vi "DrawChampionsScreen.vi"(8 "error in (no error)":errorcluster, 11 "SnakeGame in":refnum<class "SnakeGame.lvclass">) -> (0 "error out":errorcluster, 3 "SnakeGame out":refnum<class "SnakeGame.lvclass">)   [LabVIEW 2019, in "RT_Game.lvlib" / "SnakeGame.lvclass"]
uses:
  SnakeGame.lvclass
  Engine/Engine.lvclass
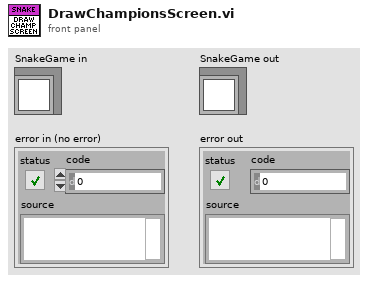
[diagram p1: front panel]
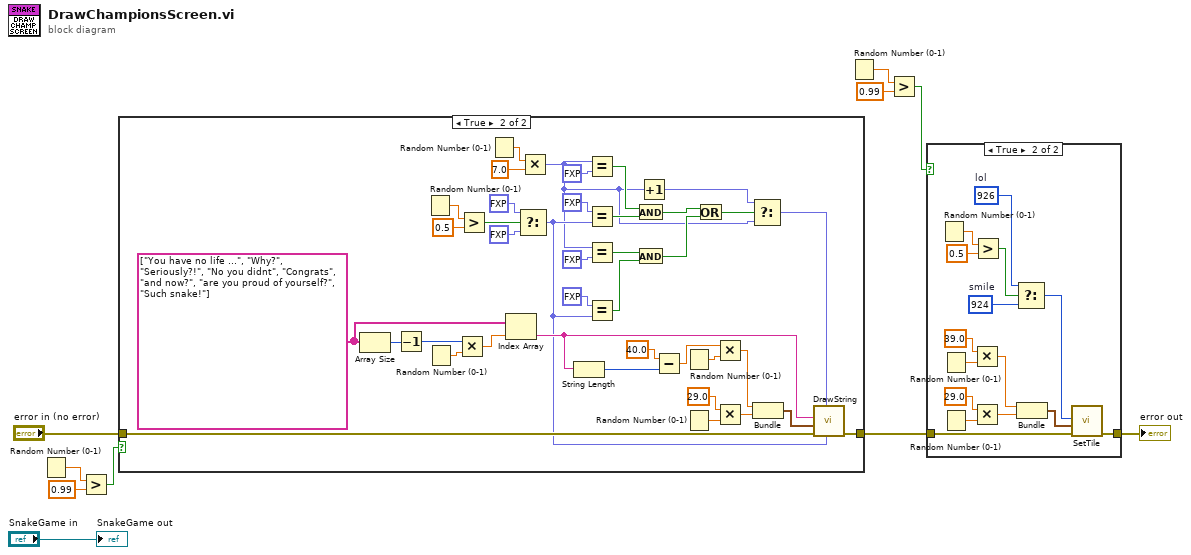
[diagram p0: block diagram]
diagram:
  n1 = Random Number (0-1)() -> (number: 0 to 1=w3:dbl)
  n2 = Greater?(x=w3, y=0.99) -> (0:w4:bool)
  n3 = case shown="True" w4 {
    tunnel: "error in (no error)" -> [w11 w50]
    tunnel: [w11 w27] -> w7
    frame False {
    }
    frame True {
      w49 = string[] ["You have no life ...", "Why?", "Seriously?!", "No you didnt", "Congrats", "and now?", "are you proud of yourself?", "Such snake!"]
      n4 = Array Size(array=w49) -> (size(s)=w48:i32)
      n5 = Decrement(x=w48) -> (x-1=w45:i32)
      n6 = Random Number (0-1)() -> (number: 0 to 1=w32:dbl)
      n7 = Random Number (0-1)() -> (number: 0 to 1=w47:dbl)
      n8 = Multiply(x=w45, y=w47) -> (x*y=w46:dbl)
      n9 = Greater?(x=w32, y=0.5) -> (0:w28:bool)
      n10 = Random Number (0-1)() -> (number: 0 to 1=w34:dbl)
      n11 = Index Array(array=w49, index=w46) -> (element=w44:string)
      n12 = Select(t=fxp<+,3,3> 0.0, s=w28, f=fxp<+,3,3> 7.0 ("ColorToReplace (7=white)")) -> (s? t:f=w18:fxp<+,3,3>)
      n13 = Multiply(x=w34, y=7.0) -> (x*y=w13:fxp<+,3,3>)
      n14 = String Length(string=w44) -> (length=w42:i32)
      n15 = Equal?(x=w13, y=fxp<+,3,3> 7.0) -> (x = y?=w24:bool)
      n16 = Equal?(x=fxp<+,3,3> 0.0 ("y"), y=w18) -> (x = y?=w23:bool)
      n17 = Equal?(x=w13, y=fxp<+,3,3> 0.0) -> (x = y?=w21:bool)
      n18 = Equal?(x=fxp<+,3,3> 7.0 ("y"), y=w18) -> (x = y?=w22:bool)
      n19 = And(x=w24, y=w23) -> (x .and. y?=w16:bool)
      n20 = And(x=w21, y=w22) -> (x .and. y?=w17:bool)
      n21 = Increment(x=w13) -> (x+1=w14:fxp<+,3,3>)
      n22 = Subtract(x=40.0, y=w42) -> (x-y=w40:dbl)
      n23 = Random Number (0-1)() -> (number: 0 to 1=w41:dbl)
      n24 = Random Number (0-1)() -> (number: 0 to 1=w38:dbl)
      n25 = Or(x=w16, y=w17) -> (x .or. y?=w12:bool)
      n26 = Multiply(x=w40, y=w41) -> (x*y=w39:dbl)
      n27 = Multiply(x=29.0, y=w38) -> (x*y=w36:dbl)
      n28 = Select(t=w14, s=w12, f=w13) -> (s? t:f=w15:fxp<+,3,3>)
      n29 = Bundle(w39, w36) -> (w35:cluster{dbl, dbl})  [unwired: 1 in]
      n30 = call "DrawString.vi"("ColorToReplace (7=white)"=w18, "Color (7=white)"=w15, "error in (no error)"=w50, "Coordinate"=w35, "String"=w44) -> ("error out"=w27:errorcluster)  [unwired: 6 in]
    }
  }
  n31 = Random Number (0-1)() -> (number: 0 to 1=w9:dbl)
  n32 = Greater?(x=w9, y=0.99) -> (0:w10:bool)
  n33 = case shown="True" w10 {
    tunnel: [w51 w59] -> w6
    tunnel: w7 -> [w51 w58]
    frame False {
    }
    frame True {
      w53 = u32 924  # smile
      w54 = u32 926  # lol
      n34 = Random Number (0-1)() -> (number: 0 to 1=w56:dbl)
      n35 = Random Number (0-1)() -> (number: 0 to 1=w64:dbl)
      n36 = Random Number (0-1)() -> (number: 0 to 1=w62:dbl)
      n37 = Multiply(x=39.0, y=w64) -> (x*y=w63:dbl)
      n38 = Multiply(x=29.0, y=w62) -> (x*y=w65:dbl)
      n39 = Greater?(x=w56, y=0.5) -> (0:w52:bool)
      n40 = Select(t=w54, s=w52, f=w53) -> (s? t:f=w55:u32)
      n41 = Bundle(w63, w65) -> (w66:cluster{dbl, dbl})  [unwired: 1 in]
      n42 = call "SetTile.vi"("error in (no error)"=w58, "Coordinates"=w66, "TileCode"=w55) -> ("error out"=w59:errorcluster)  [unwired: 8 in]
    }
  }
  "error out" <- w6
  "SnakeGame out" <- "SnakeGame in"
